vi "Send Message Normal Check.vi"(4 "Source (\"\")":string, 6 "Timeout (25000)":u32=25000, 8 "error in (no error)":errorcluster, 10 "Send Message (\"\")":string, 11 "VISA resource name":refnum<visa-resource-name>) -> (0 "error out":errorcluster, 1 "Read Buffer@":string, 2 "Response Type":i32(ring) items=["Affirmative", "Single Negative", "Multiple Negative", "ASCII", "Binary", "End"], 3 "VISA resource name out":refnum<visa-resource-name>, 5 "Internal Error Number":i32 max=999 step=1, 7 "Internal Error String":string)   [LabVIEW 2011, in "Yokogawa DX Series.lvlib"]
doc: "This VI sends the message. Then it returns the response and checks the message.\nThen this returns Internal Error Type. If the message is an error message, this sets \"command are not processed succesfully\" to error out."
uses:
  <instrlib>/Yokogawa DX Series/Yokogawa DX Series.lvlib
panel:
  # "msec"
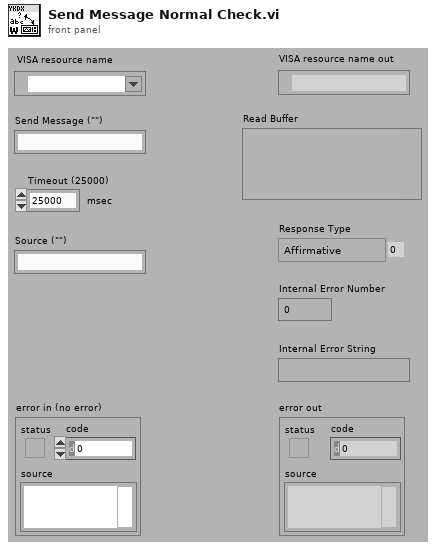
[diagram p1: front panel]
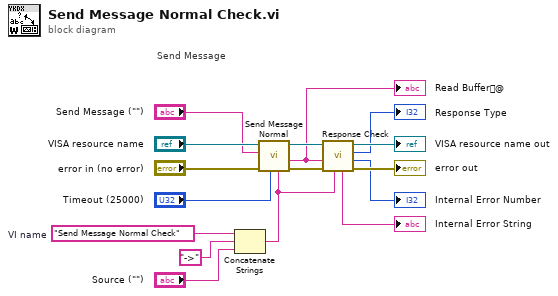
[diagram p0: block diagram]
diagram:
  w16 = "Send Message Normal Check"  # VI name
  # "Send Message"
  n1 = Concatenate Strings(w16, "->", "Source (\"\")") -> (w7:string)
  n2 = call <instrlib>:"Send Message Normal.vi"("Source (\"\")"=w7, "Timeout (25000)"="Timeout (25000)", "error in (no error)"="error in (no error)", "Send Message (\"\")"="Send Message (\"\")", "VISA resource name"="VISA resource name") -> ("error out"=w8:errorcluster, "Read Buffer"=w1:string, "VISA resource name out"=w9:refnum<visa-resource-name>)  [unwired: 4 out]
  "Read Buffer@" <- w1
  n3 = call <instrlib>:"Response Check.vi"("Source (\"\")"=w7, "error in (no error)"=w8, "Message In (\"\")"=w1, "VISA resource name"=w9) -> ("error out"=→"error out":errorcluster, "Internal Error Number"=→"Internal Error Number":i32, "Response Type"=→"Response Type":i32, "VISA resource name out"=→"VISA resource name out":refnum<visa-resource-name>, "Internal Error String"=→"Internal Error String":string)  [unwired: 3 out]
